vi "Table Color Update.vi"(9 "Value":string[][](array[string]), 10 "Current Step ID":i32, 11 "Test Table":refnum<vi>) -> ()   [LabVIEW 2018]
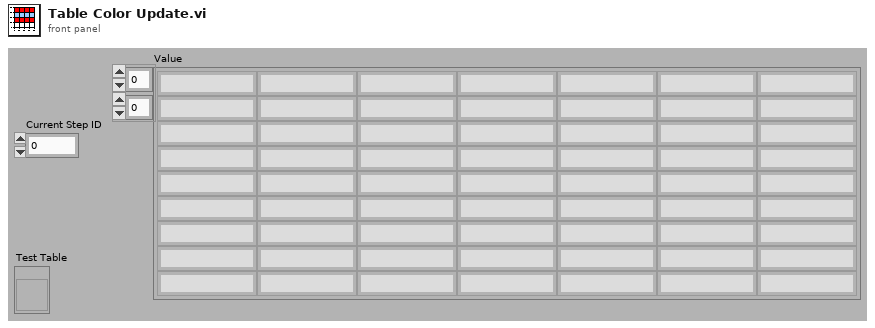
[diagram p1: front panel]
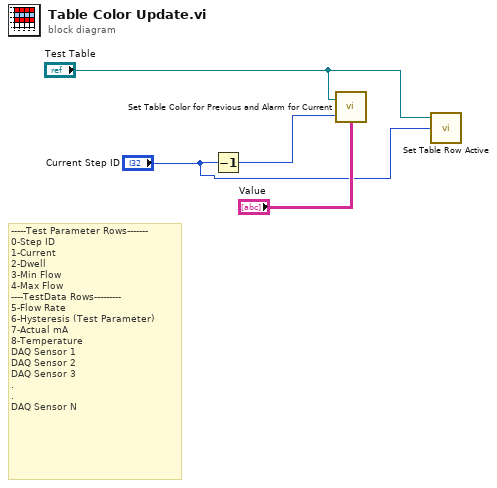
[diagram p0: block diagram]
diagram:
  # "-----Test Parameter Rows-------\n0-Step ID\n1-Current\n2-Dwell\n3-Min Flow\n4-Max Flow\n----TestData Rows---------\n5-Flow Rate\n6-Hysteresis (Test Parameter)\n7-Actual mA\n8-Temperature\nDAQ Sensor 1\nDAQ Sensor 2\nDAQ Sensor 3\n.\n.\nDAQ Sensor N"
  n1 = Decrement(x="Current Step ID") -> (x-1=w2:i32)
  n2 = call "Set Table Color for Previous and Alarm for Current.vi"("Test Table"="Test Table", "Previous Step ID"=w2, "Value"="Value") -> ()  [unwired: 13 in]
  n3 = call "Set Table Row Active.vi"("Current Step ID"="Current Step ID", "Test Table"="Test Table") -> ()  [unwired: 1 in]
